vi "Lookup Base Protocol Class and Info.vi"(8 "error in (no error)":errorcluster, 10 "Protocol in":string, 11 "Class Lookup":variant) -> (0 "error out":errorcluster, 1 "Protocol out":T1, 2 "Protocol Parent out":refnum<class "Protocol Parent.lvclass">, 3 "Class Lookup out":variant, 4 "Error Codes":cluster{"Code":i32, "String":string}[](array[cluster]))   [LabVIEW 2018, in "Protocols.lvlib"]
uses:
  Protocols.lvlib
  Protocol Parent.lvclass
  Types/Base Protocol Type.ctl
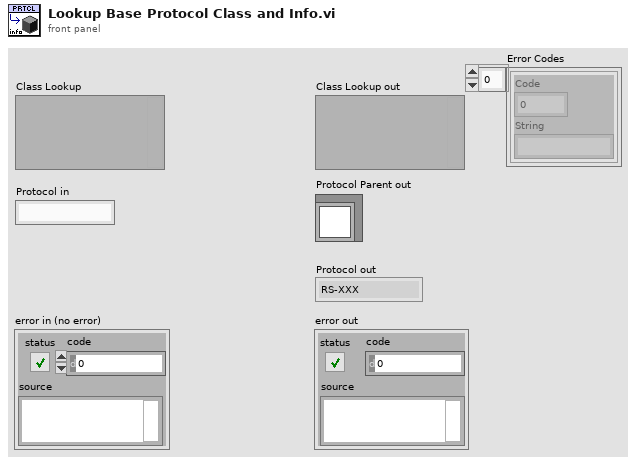
[diagram p1: front panel]
types:
  T1 = typedef "Protocols.lvlib/Protocol Parent.lvclass/Base Protocol Type.ctl" = enum16{"RS-XXX", "VISA", "TCPIP", "UDP", "GPIB ConvBox"}
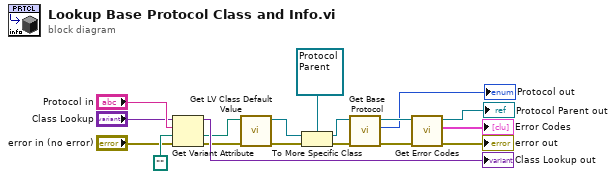
[diagram p0: block diagram]
diagram:
  n1 = Get Variant Attribute(Variant="Class Lookup", name="Protocol in", default value (empty Variant)=path "", error in="error in (no error)") -> (duplicate Variant=→"Class Lookup out":variant, value=w12:path, error out=w13:errorcluster)  [unwired: 1 out]
  n2 = call <vilib>:"Get LV Class Default Value.vi"("error in (no error)"=w13, "class path"=w12) -> ("error out"=w14:errorcluster, "object"=w16:refnum<class>)  [unwired: 8 in]
  n3 = To More Specific Class(target class=refnum<class "Protocol Parent.lvclass"> refnum ("Protocols.lvlib:Protocol Parent.lvclass"), reference=w16, error in=w14) -> (specific class reference=w17:refnum<class "Protocol Parent.lvclass">, error out=w15:errorcluster)
  n4 = call-dynamic "Get Base Protocol.vi"("error in (no error)"=w15, "Protocol Parent in"=w17) -> ("error out"=w7:errorcluster, "Protocol out"=→"Protocol out":T1, "Protocol Parent out"=w6:refnum<class "Protocol Parent.lvclass">)  [unwired: 7 in]
  n5 = call-dynamic "Get Error Codes.vi"("error in (no error)"=w7, "Protocol Parent in"=w6) -> ("error out"=→"error out":errorcluster, "Error Codes"=→"Error Codes":cluster{"Code":i32, "String":string}[], "Protocol Parent out"=→"Protocol Parent out":refnum<class "Protocol Parent.lvclass">)  [unwired: 7 in]
